vi "Bemeneti_parameterek.vi"(10 "Parameterek":T1={"rholevego"=1.3, "Vlevego"=0.446, "Mlevego"=0.0, "clevego"=1.0, "rho PCM"=1100.0, "rho kulso"=28.3, "Dkulso"=0.1, "nkulso"=10, "dkulso"=0.0, "vkulso"=0.0, "rho kozepso"=28.3, "Dkozepso"=0.06, "nkozepso"=6, "dkozepso"=0.0, "vkozepso"=0.0, "mkozepso"=0.0, "mkulso"=0.0, "rho belso"=28.3, "Dbelso"=0.1, "nbelso"=10, "dbelso"=0.0, "vbelso"=0.0, "mbelso"=0.0, "Xpcm_kulso"=0.3, "Xpcm_belso"=0.3, "mpcm_kulso"=0.0, "mpcm_belso"=0.0, "mkulso_pcm"=0.0, "mbelso_pcm"=0.0, "ckulso"=1.13, "ckozepso"=1.13, "cbelso"=1.13, "cpcm_szilard"=1.9, "cpcm_foly"=1.5, "ckulso_Topalatt"=0.0, "cbelso_Topalatt"=0.0, "ckulso_Topfelett"=0.0, "cbelso_Topfelett"=0.0, "hpcm_olv"=140.0, "ckulso_eff_Tolv"=0.0, "cbelso_eff_Tolv"=0.0, "Qkulso_op_also"=0.0, "Qkulso_op_felso"=0.0, "Qbelso_op_also"=0.0, "Qbelso_op_felso"=0.0, "lambda_kulso"=5e-05, "lambda_kozepso"=5e-05, "lambda_belso"=5e-05, "lambda_pcm"=0.00018, "VXpcm_kulso"=0.0, "VXpcm_belso"=0.0, "lambda_kulsoPCM"=0.0, "lambda_belsoPCM"=0.0, "Alfa_kulso"=0.015, "Alfa_belso"=0.006, "Alfa_kont"=0.03, "Top_also"=24.0, "Top_felso"=28.0, "cpcm_olvnelkul"=1.0, "Tbelsolevego_0"=22.0}) -> (2 "Parameterek 2":T1={"rholevego"=0.0, "Vlevego"=0.0, "Mlevego"=0.0, "clevego"=0.0, "rho PCM"=1100.0, "rho kulso"=28.3, "Dkulso"=0.1, "nkulso"=10, "dkulso"=0.0, "vkulso"=0.0, "rho kozepso"=28.3, "Dkozepso"=0.06, "nkozepso"=6, "dkozepso"=0.0, "vkozepso"=0.0, "mkozepso"=0.0, "mkulso"=0.0, "rho belso"=28.3, "Dbelso"=0.1, "nbelso"=10, "dbelso"=0.0, "vbelso"=0.0, "mbelso"=0.0, "Xpcm_kulso"=0.3, "Xpcm_belso"=0.3, "mpcm_kulso"=0.0, "mpcm_belso"=0.0, "mkulso_pcm"=0.0, "mbelso_pcm"=0.0, "ckulso"=1.13, "ckozepso"=1.13, "cbelso"=1.13, "cpcm_szilard"=1.9, "cpcm_foly"=1.5, "ckulso_Topalatt"=0.0, "cbelso_Topalatt"=0.0, "ckulso_Topfelett"=0.0, "cbelso_Topfelett"=0.0, "hpcm_olv"=140.0, "ckulso_eff_Tolv"=0.0, "cbelso_eff_Tolv"=0.0, "Qkulso_op_also"=0.0, "Qkulso_op_felso"=0.0, "Qbelso_op_also"=0.0, "Qbelso_op_felso"=0.0, "lambda_kulso"=5e-05, "lambda_kozepso"=5e-05, "lambda_belso"=5e-05, "lambda_pcm"=0.00018, "VXpcm_kulso"=0.0, "VXpcm_belso"=0.0, "lambda_kulsoPCM"=0.0, "lambda_belsoPCM"=0.0, "Alfa_kulso"=0.015, "Alfa_belso"=0.006, "Alfa_kont"=0.03, "Top_also"=24.0, "Top_felso"=28.0, "cpcm_olvnelkul"=0.0, "Tbelsolevego_0"=22.0})   [LabVIEW 2013]
uses:
  Parameterek.ctl
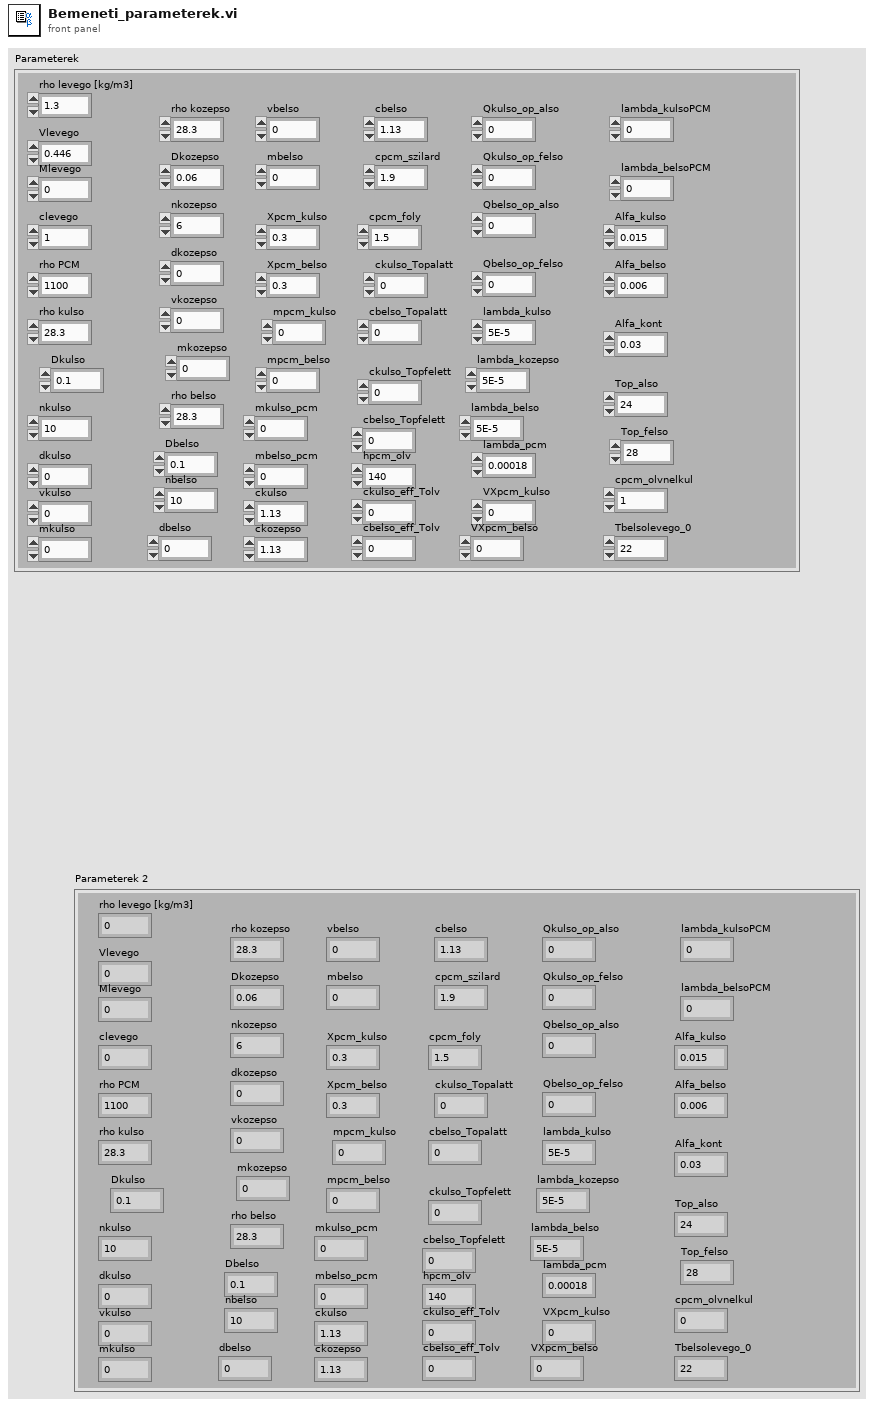
[diagram p1: front panel]
types:
  T1 = typedef "Parameterek.ctl" = cluster{"rholevego":dbl, "Vlevego":dbl, "Mlevego":dbl, "clevego":dbl, "rho PCM":dbl, "rho kulso":dbl, "Dkulso":dbl, "nkulso":i32, "dkulso":dbl, "vkulso":dbl, "rho kozepso":dbl, "Dkozepso":dbl, "nkozepso":i32, "dkozepso":dbl, "vkozepso":dbl, "mkozepso":dbl, "mkulso":dbl, "rho belso":dbl, "Dbelso":dbl, "nbelso":i32, "dbelso":dbl, "vbelso":dbl, "mbelso":dbl, "Xpcm_kulso":dbl, "Xpcm_belso":dbl, "mpcm_kulso":dbl, "mpcm_belso":dbl, "mkulso_pcm":dbl, "mbelso_pcm":dbl, "ckulso":dbl, "ckozepso":dbl, "cbelso":dbl, "cpcm_szilard":dbl, "cpcm_foly":dbl, "ckulso_Topalatt":dbl, "cbelso_Topalatt":dbl, "ckulso_Topfelett":dbl, "cbelso_Topfelett":dbl, "hpcm_olv":dbl, "ckulso_eff_Tolv":dbl, "cbelso_eff_Tolv":dbl, "Qkulso_op_also":dbl, "Qkulso_op_felso":dbl, "Qbelso_op_also":dbl, "Qbelso_op_felso":dbl, "lambda_kulso":dbl, "lambda_kozepso":dbl, "lambda_belso":dbl, "lambda_pcm":dbl, "VXpcm_kulso":dbl, "VXpcm_belso":dbl, "lambda_kulsoPCM":dbl, "lambda_belsoPCM":dbl, "Alfa_kulso":dbl, "Alfa_belso":dbl, "Alfa_kont":dbl, "Top_also":dbl, "Top_felso":dbl, "cpcm_olvnelkul":dbl, "Tbelsolevego_0":dbl}
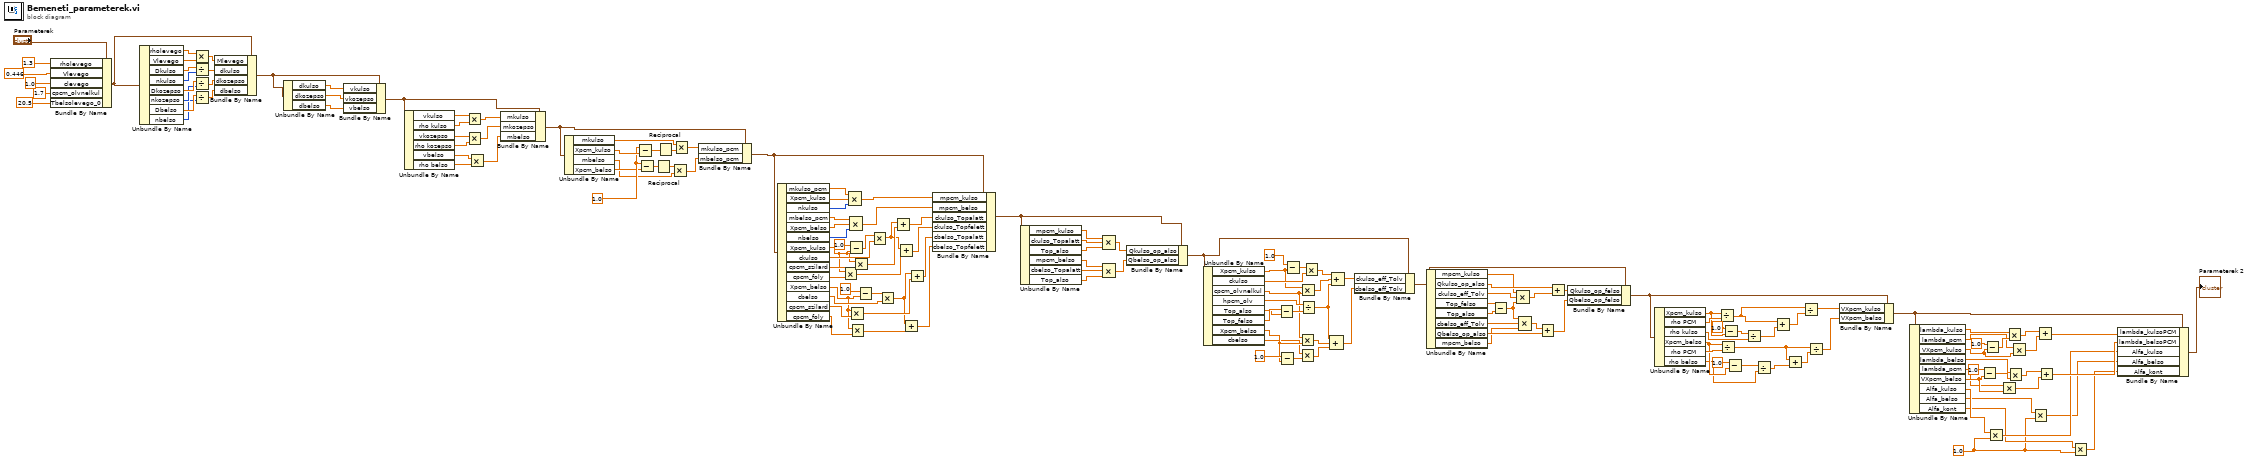
[diagram p0: block diagram]
diagram:
  w10 = 1.0 ("y")
  w130 = 1.0
  n1 = Bundle By Name(cluster="Parameterek", "rholevego"=1.3, "Vlevego"=0.446, "clevego"=1.0, "cpcm_olvnelkul"=1.7, "Tbelsolevego_0"=20.5) -> (w17:T1)
  n2 = Unbundle By Name(w17) -> ("rholevego"=w164:dbl, "Vlevego"=w163:dbl, "Dkulso"=w161:dbl, "nkulso"=w160:i32, "Dkozepso"=w158:dbl, "nkozepso"=w157:i32, "Dbelso"=w155:dbl, "nbelso"=w154:i32)
  n3 = Multiply(x=w164, y=w163) -> (x*y=w162:dbl)
  n4 = Divide(x=w161, y=w160) -> (x/y=w159:dbl)
  n5 = Divide(x=w158, y=w157) -> (x/y=w156:dbl)
  n6 = Divide(x=w155, y=w154) -> (x/y=w153:dbl)
  n7 = Bundle By Name(cluster=w17, "Mlevego"=w162, "dkulso"=w159, "dkozepso"=w156, "dbelso"=w153) -> (w152:T1)
  n8 = Unbundle By Name(w152) -> ("dkulso"=w151:dbl, "dkozepso"=w150:dbl, "dbelso"=w149:dbl)
  n9 = Bundle By Name(cluster=w152, "vkulso"=w151, "vkozepso"=w150, "vbelso"=w149) -> (w148:T1)
  n10 = Unbundle By Name(w148) -> ("vkulso"=w147:dbl, "rho kulso"=w146:dbl, "vkozepso"=w142:dbl, "rho kozepso"=w141:dbl, "vbelso"=w140:dbl, "rho belso"=w139:dbl)
  n11 = Multiply(x=w147, y=w146) -> (x*y=w145:dbl)
  n12 = Multiply(x=w142, y=w141) -> (x*y=w144:dbl)
  n13 = Multiply(x=w140, y=w139) -> (x*y=w143:dbl)
  n14 = Bundle By Name(cluster=w148, "mkulso"=w145, "mkozepso"=w144, "mbelso"=w143) -> (w138:T1)
  n15 = Unbundle By Name(w138) -> ("mkulso"=w135:dbl, "Xpcm_kulso"=w137:dbl, "mbelso"=w128:dbl, "Xpcm_belso"=w129:dbl)
  n16 = Subtract(x=w130, y=w137) -> (x-y=w133:dbl)
  n17 = Subtract(x=w130, y=w129) -> (x-y=w132:dbl)
  n18 = Reciprocal(x=w132) -> (1/x=w131:dbl)
  n19 = Reciprocal(x=w133) -> (1/x=w136:dbl)
  n20 = Multiply(x=w131, y=w128) -> (x*y=w127:dbl)
  n21 = Multiply(x=w135, y=w136) -> (x*y=w134:dbl)
  n22 = Bundle By Name(cluster=w138, "mkulso_pcm"=w134, "mbelso_pcm"=w127) -> (w125:T1)
  n23 = Unbundle By Name(w125) -> ("mkulso_pcm"=w124:dbl, "Xpcm_kulso"=w123:dbl, "nkulso"=w122:i32, "mbelso_pcm"=w121:dbl, "Xpcm_belso"=w120:dbl, "nbelso"=w119:i32, "Xpcm_kulso"=w110:dbl, "ckulso"=w115:dbl, "cpcm_szilard"=w114:dbl, "cpcm_foly"=w111:dbl, "Xpcm_belso"=w99:dbl, "cbelso"=w104:dbl, "cpcm_szilard"=w103:dbl, "cpcm_foly"=w100:dbl)
  n24 = Multiply(x=w110, y=w111) -> (x*y=w109:dbl)
  n25 = Subtract(x=1.0, y=w110) -> (x-y=w116:dbl)
  n26 = Multiply(x=w99, y=w103) -> (x*y=w102:dbl)
  n27 = Compound Arithmetic op=MULTIPLY(w124, w123, w122) -> (w126:dbl)
  n28 = Multiply(x=w99, y=w100) -> (x*y=w98:dbl)
  n29 = Compound Arithmetic op=MULTIPLY(w121, w120, w119) -> (w118:dbl)
  n30 = Multiply(x=w110, y=w114) -> (x*y=w113:dbl)
  n31 = Subtract(x=1.0, y=w99) -> (x-y=w105:dbl)
  n32 = Multiply(x=w116, y=w115) -> (x*y=w108:dbl)
  n33 = Multiply(x=w105, y=w104) -> (x*y=w97:dbl)
  n34 = Add(x=w108, y=w113) -> (x+y=w112:dbl)
  n35 = Add(x=w108, y=w109) -> (x+y=w107:dbl)
  n36 = Add(x=w97, y=w98) -> (x+y=w96:dbl)
  n37 = Add(x=w97, y=w102) -> (x+y=w101:dbl)
  n38 = Bundle By Name(cluster=w125, "mpcm_kulso"=w126, "mpcm_belso"=w118, "ckulso_Topalatt"=w112, "ckulso_Topfelett"=w107, "cbelso_Topalatt"=w101, "cbelso_Topfelett"=w96) -> (w95:T1)
  n39 = Unbundle By Name(w95) -> ("mpcm_kulso"=w94:dbl, "ckulso_Topalatt"=w93:dbl, "Top_also"=w92:dbl, "mpcm_belso"=w90:dbl, "cbelso_Topalatt"=w89:dbl, "Top_also"=w88:dbl)
  n40 = Compound Arithmetic op=MULTIPLY(w94, w93, w92) -> (w91:dbl)
  n41 = Compound Arithmetic op=MULTIPLY(w90, w89, w88) -> (w87:dbl)
  n42 = Bundle By Name(cluster=w95, "Qkulso_op_also"=w91, "Qbelso_op_also"=w87) -> (w86:T1)
  n43 = Unbundle By Name(w86) -> ("Xpcm_kulso"=w81:dbl, "ckulso"=w83:dbl, "cpcm_olvnelkul"=w74:dbl, "hpcm_olv"=w77:dbl, "Top_also"=w78:dbl, "Top_felso"=w79:dbl, "Xpcm_belso"=w70:dbl, "cbelso"=w68:dbl)
  n44 = Subtract(x=w79, y=w78) -> (x-y=w76:dbl)
  n45 = Subtract(x=1.0, y=w70) -> (x-y=w69:dbl)
  n46 = Subtract(x=1.0, y=w81) -> (x-y=w84:dbl)
  n47 = Multiply(x=w74, y=w70) -> (x*y=w73:dbl)
  n48 = Multiply(x=w68, y=w69) -> (x*y=w67:dbl)
  n49 = Multiply(x=w81, y=w74) -> (x*y=w80:dbl)
  n50 = Divide(x=w77, y=w76) -> (x/y=w72:dbl)
  n51 = Multiply(x=w84, y=w83) -> (x*y=w82:dbl)
  n52 = Compound Arithmetic op=ADD(w72, w73, w67) -> (w66:dbl)
  n53 = Compound Arithmetic op=ADD(w82, w80, w72) -> (w75:dbl)
  n54 = Bundle By Name(cluster=w86, "ckulso_eff_Tolv"=w75, "cbelso_eff_Tolv"=w66) -> (w65:T1)
  n55 = Unbundle By Name(w65) -> ("mpcm_kulso"=w6:dbl, "Qkulso_op_also"=w63:dbl, "ckulso_eff_Tolv"=w7:dbl, "Top_felso"=w62:dbl, "Top_also"=w61:dbl, "cbelso_eff_Tolv"=w3:dbl, "Qbelso_op_also"=w60:dbl, "mpcm_belso"=w2:dbl)
  n56 = Subtract(x=w62, y=w61) -> (x-y=w4:dbl)
  n57 = Compound Arithmetic op=MULTIPLY(w6, w7, w4) -> (w5:dbl)
  n58 = Compound Arithmetic op=MULTIPLY(w4, w3, w2) -> (w1:dbl)
  n59 = Add(x=w1, y=w60) -> (x+y=w59:dbl)
  n60 = Add(x=w63, y=w5) -> (x+y=w64:dbl)
  n61 = Bundle By Name(cluster=w65, "Qkulso_op_felso"=w64, "Qbelso_op_felso"=w59) -> (w58:T1)
  n62 = Unbundle By Name(w58) -> ("Xpcm_kulso"=w53:dbl, "rho PCM"=w57:dbl, "rho kulso"=w51:dbl, "Xpcm_belso"=w45:dbl, "rho PCM"=w47:dbl, "rho belso"=w40:dbl)
  n63 = Divide(x=w53, y=w57) -> (x/y=w55:dbl)
  n64 = Divide(x=w45, y=w47) -> (x/y=w43:dbl)
  n65 = Subtract(x=1.0, y=w53) -> (x-y=w52:dbl)
  n66 = Subtract(x=1.0, y=w45) -> (x-y=w41:dbl)
  n67 = Divide(x=w52, y=w51) -> (x/y=w50:dbl)
  n68 = Divide(x=w41, y=w40) -> (x/y=w42:dbl)
  n69 = Add(x=w55, y=w50) -> (x+y=w49:dbl)
  n70 = Add(x=w43, y=w42) -> (x+y=w44:dbl)
  n71 = Divide(x=w55, y=w49) -> (x/y=w56:dbl)
  n72 = Divide(x=w43, y=w44) -> (x/y=w48:dbl)
  n73 = Bundle By Name(cluster=w58, "VXpcm_kulso"=w56, "VXpcm_belso"=w48) -> (w39:T1)
  n74 = Unbundle By Name(w39) -> ("lambda_kulso"=w35:dbl, "lambda_pcm"=w30:dbl, "VXpcm_kulso"=w31:dbl, "lambda_belso"=w25:dbl, "lambda_pcm"=w24:dbl, "VXpcm_belso"=w27:dbl, "Alfa_kulso"=w16:dbl, "Alfa_belso"=w14:dbl, "Alfa_kont"=w12:dbl)
  n75 = Subtract(x=1.0, y=w27) -> (x-y=w26:dbl)
  n76 = Subtract(x=1.0, y=w31) -> (x-y=w36:dbl)
  n77 = Multiply(x=w16, y=w10) -> (x*y=w15:dbl)
  n78 = Multiply(x=w24, y=w27) -> (x*y=w22:dbl)
  n79 = Multiply(x=w35, y=w36) -> (x*y=w34:dbl)
  n80 = Multiply(x=w25, y=w26) -> (x*y=w23:dbl)
  n81 = Multiply(x=w30, y=w31) -> (x*y=w29:dbl)
  n82 = Multiply(x=w14, y=w10) -> (x*y=w13:dbl)
  n83 = Add(x=w34, y=w29) -> (x+y=w33:dbl)
  n84 = Add(x=w23, y=w22) -> (x+y=w32:dbl)
  n85 = Multiply(x=w12, y=w10) -> (x*y=w11:dbl)
  n86 = Bundle By Name(cluster=w39, "lambda_kulsoPCM"=w33, "lambda_belsoPCM"=w32, "Alfa_kulso"=w15, "Alfa_belso"=w13, "Alfa_kont"=w11) -> (→"Parameterek 2":T1)
